vi "trapezoidal_generica.vi"(11 "Slide":dbl(slide) scale=0.0..10.0) -> (3 "Waveform Pattern":dbl[](graph))   [LabVIEW 2020]
doc: "Esse VI eh responsavel por gerar uma onda com formato trapezoidal."
uses:
  <vilib>/Analysis/1siggen.llb/Ramp Pattern by Samples.vi
  <vilib>/Analysis/NI_AALBase.lvlib
panel:
  in  "Boolean":bool
  in  "Stop":bool
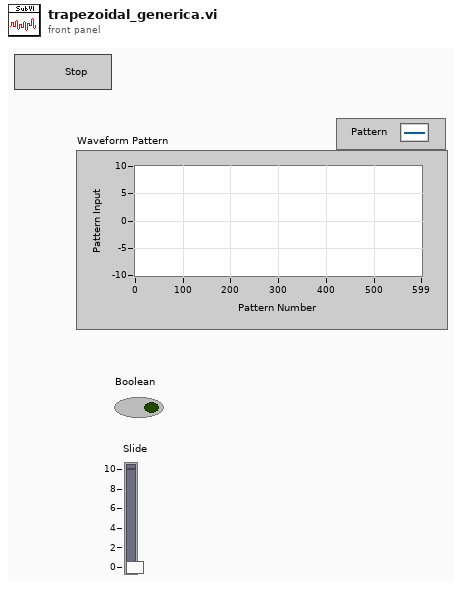
[diagram p1: front panel]
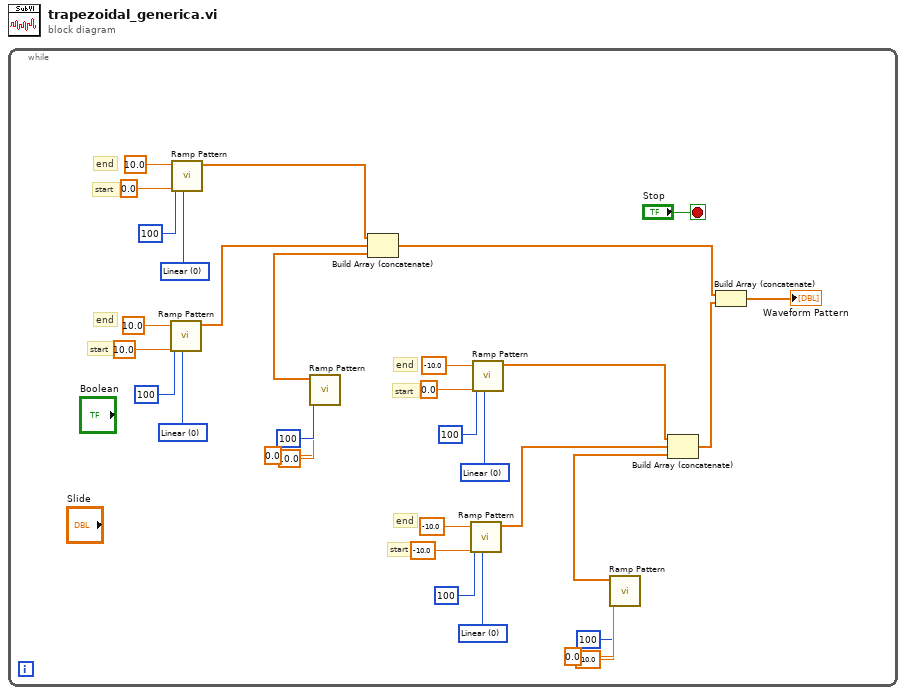
[diagram p0: block diagram]
diagram:
  n1 = while {
    stop <- "Stop" stop-if-true
    w8 = u16 0 items=["Linear", "Logarithmic"] ("type")
    w4 = u16 0 items=["Linear", "Logarithmic"] ("type")
    w27 = u16 0 items=["Linear", "Logarithmic"] ("type")
    w31 = u16 0 items=["Linear", "Logarithmic"] ("type")
    # "start"
    # "end"
    # "end"
    # "start"
    # "start"
    # "end"
    # "end"
    # "start"
    n2 = call-poly <vilib>:"Ramp Pattern.vi"("type"=w27, "start"=10.0, "end"=10.0, "samples"=100) -> ("Ramp Pattern"=w23:dbl[])  [unwired: 6 in, 1 out]
    n3 = call-poly <vilib>:"Ramp Pattern.vi"("type"=w31, "start"=0.0, "end"=10.0, "samples"=100) -> ("Ramp Pattern"=w22:dbl[])  [unwired: 6 in, 1 out]
    n4 = call-poly <vilib>:"Ramp Pattern.vi"("start"=10.0, "end"=0.0, "samples"=100) -> ("Ramp Pattern"=w18:dbl[])  [unwired: 7 in, 1 out]
    n5 = Build Array (concatenate)(w22, w23, w18) -> (w3:dbl[])
    n6 = call-poly <vilib>:"Ramp Pattern.vi"("type"=w8, "start"=-10.0, "end"=-10.0, "samples"=100) -> ("Ramp Pattern"=w12:dbl[])  [unwired: 6 in, 1 out]
    n7 = call-poly <vilib>:"Ramp Pattern.vi"("type"=w4, "start"=0.0, "end"=-10.0, "samples"=100) -> ("Ramp Pattern"=w13:dbl[])  [unwired: 6 in, 1 out]
    n8 = call-poly <vilib>:"Ramp Pattern.vi"("start"=-10.0, "end"=0.0, "samples"=100) -> ("Ramp Pattern"=w17:dbl[])  [unwired: 7 in, 1 out]
    n9 = Build Array (concatenate)(w13, w12, w17) -> (w2:dbl[])
    n10 = Build Array (concatenate)(w3, w2) -> (→"Waveform Pattern":dbl[])
  }
